vi "Ensemble Empirical Mode Decomposition.vi"(5 "Ensemble Size":u32, 7 "IMF Tolerance":dbl=0.2 format="%#_13g", 11 "Waveform":waveform(dbl)) -> (0 "df":dbl, 1 "dt":dbl, 2 "Hilbert Spectra":dbl[][][](array[numeric]), 3 "IMF Array":waveform(dbl)[](array[waveform]))   [LabVIEW 2013, in "Empirical Mode Decomposition.lvlib"]
uses:
  Empirical Mode Decomposition.lvlib
  <vilib>/Waveform/WDTOps.llb/WDT Number of Waveform Samples DBL.vi
  <vilib>/measure/mascope.llb/Amplitude and Levels 1 chan.vi
  <vilib>/measure/NI_MABase.lvlib
  <vilib>/measure/NI_MAPro.lvlib
  Popup Progress Bar/Popup Progress Bar.lvlib
panel:
  out "IMF + 0":waveform(dbl)[](graph)
  out "IMF":waveform(dbl)[](graph)
  # "TODO: Smooth out the Hilbert Spectrum graph"
  # "Scale                  Index\n1                              512-1023\n2                              256-511\n3                              128-255\n4                              64-127\n5                              32-63\n6                              16-31\n7                              8-15\n8                              4-7\n9                              2-3"
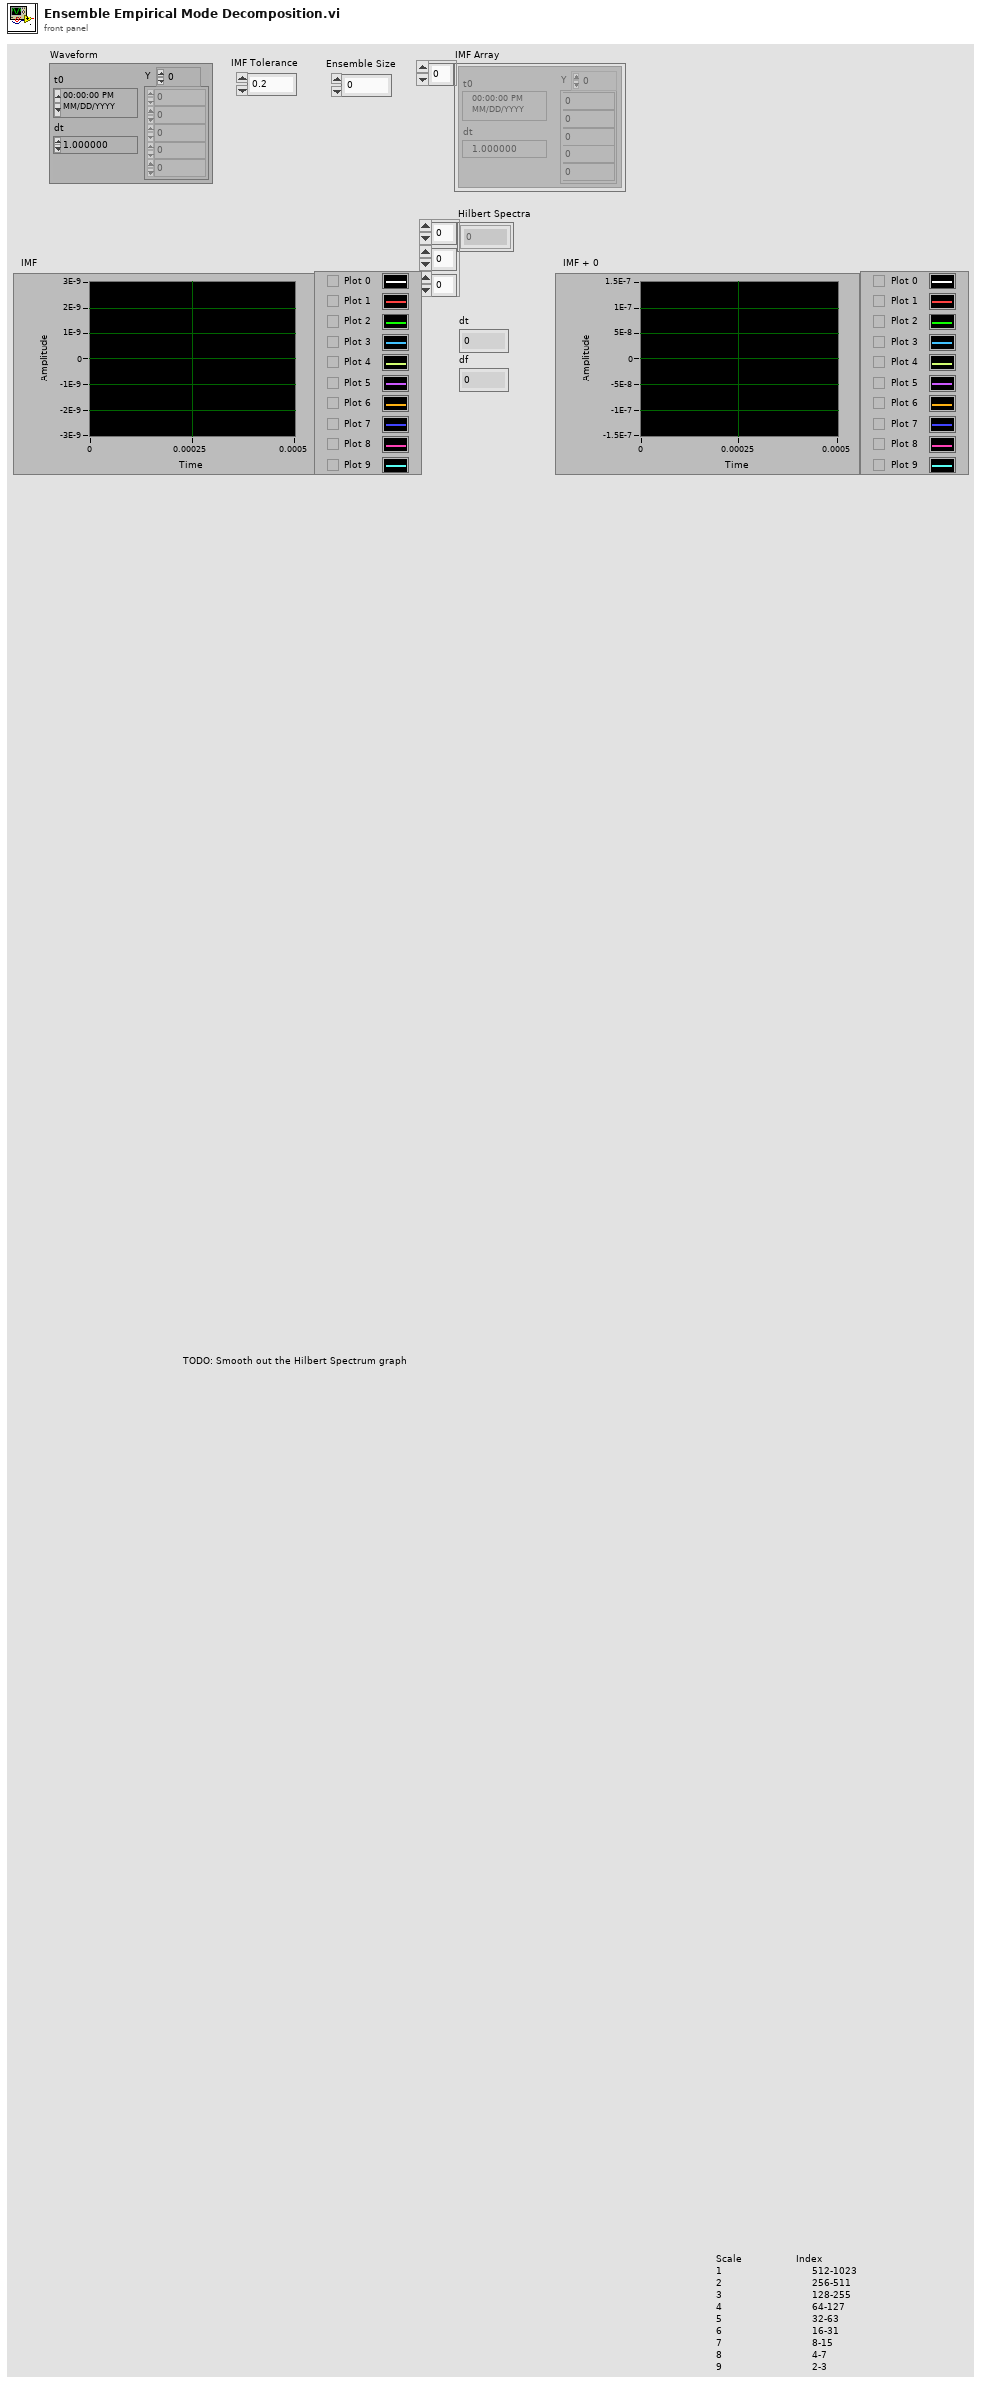
[diagram p1: front panel]
types:
  T1 = cluster{"This VI":refnum<vi>, "notifier out":refnum<notifier>}
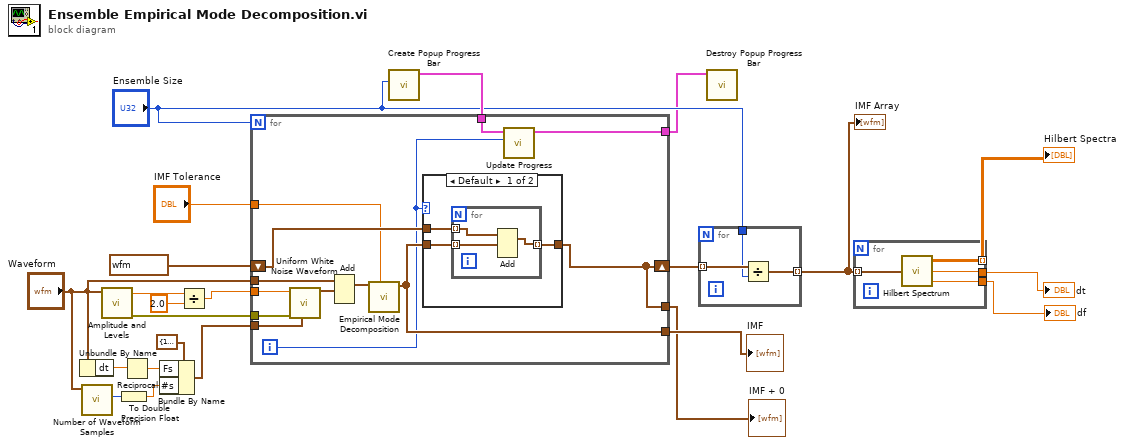
[diagram p0: block diagram]
diagram:
  n1 = Unbundle By Name("Waveform") -> ("dt"=w16:dbl)
  n2 = call-poly <vilib>:"Number of Waveform Samples.vi"("waveform in"="Waveform") -> ("number of samples"=w12:i32)  [unwired: 8 in, 2 out]
  n3 = call-poly <vilib>:"Amplitude and Levels.vi"("signal in"="Waveform") -> ("error out"=w23:errorcluster, "amplitude"=w7:dbl)  [unwired: 7 in, 2 out]
  n4 = To Double Precision Float(number=w12) -> (double precision float=w13:dbl)
  n5 = Reciprocal(x=w16) -> (1/x=w14:dbl)
  n6 = Bundle By Name(cluster=cluster{"Fs":dbl, "#s":dbl} {"Fs"=1000.0, "#s"=1000.0} ("sampling info"), "Fs"=w14, "#s"=w13) -> (w11:cluster{"Fs":dbl, "#s":dbl})
  n7 = Divide(x=w7, y=2.0) -> (x/y=w5:dbl)
  n8 = call "Create Popup Progress Bar.vi"("100% Value (100)"="Ensemble Size") -> ("bar ref"=w3:T1)  [unwired: 9 in, 1 out]
  n9 = for {
    N: "Ensemble Size" -> [_]
    tunnel: w5 -> [w36]
    tunnel: w23 -> [w35]
    tunnel: "Waveform" -> [w33]
    shift-right: [w28] -> w21
    shift-left: waveform(dbl)[] [{"t0"=timestamp(3516206484.2410417 s since 1904-01-01), "dt"=2e-12, "Y"=array[251 elements]}, {"t0"=timestamp(3516206484.2410417 s since 1904-01-01), "dt"=2e-12, "Y"=array[251 elements]}, {"t0"=timestamp(3516206484.2410417 s since 1904-01-01), "dt"=2e-12, "Y"=array[251 elements]}] ("IMF Array") -> [w29]
    tunnel: w11 -> [w31]
    tunnel: [w28] -> w8
    tunnel: [w30] -> w9
    tunnel: "IMF Tolerance" -> [w27]
    tunnel: w3 -> [w26]
    tunnel: [w24] -> w1
    i -> [w25]
    n10 = call <vilib>:"Uniform White Noise Waveform.vi"("sampling info"=w31, "error in (no error)"=w35, "amplitude"=w36) -> ("signal out"=w34:waveform(dbl))  [unwired: 7 in, 1 out]
    n11 = Add(1:w34, 2:w33) -> (0:w32:waveform(dbl))  [unwired: 1 in, 1 out]
    n12 = call "Empirical Mode Decomposition.vi"("IMF Tolerance"=w27, "Waveform"=w32) -> ("IMF Array"=w30:waveform(dbl)[])  [unwired: 6 in, 3 out]
    n13 = case shown="Default" w25 {
      tunnel: w30 -> [w39 w43]
      tunnel: [w37 w43] -> w28
      tunnel: w29 -> [w38 _]
      frame Default {
        n14 = for {
          tunnel: w39 -> [w41] mode=indexing
          tunnel: w38 -> [w42] mode=indexing
          tunnel: [w40] -> w37 mode=indexing
          n15 = Add(1:w41, 2:w42) -> (0:w40:waveform(dbl))  [unwired: 1 in, 1 out]
        }
      }
      frame 0 {
      }
    }
    n16 = call "Update Progress.vi"("Value"=w25, "bar ref in"=w26) -> ("bar ref out"=w24:T1)  [unwired: 8 in, 1 out]
  }
  "IMF" <- w9
  "IMF + 0" <- w8
  n17 = for {
    tunnel: w21 -> [w46] mode=indexing
    tunnel: [w45] -> w20 mode=indexing
    tunnel: "Ensemble Size" -> [w44]
    n18 = Divide(x=w46, y=w44) -> (x/y=w45:waveform(dbl))
  }
  "IMF Array" <- w20
  n19 = call "Destroy Popup Progress Bar.vi"("bar ref"=w1) -> ()  [unwired: 10 in, 1 out]
  n20 = for {
    tunnel: w20 -> [w50] mode=indexing
    tunnel: [w49] -> w19 mode=indexing
    tunnel: [w48] -> w18
    tunnel: [w47] -> w17
    n21 = call "Hilbert Spectrum.vi"("Waveform"=w50) -> ("df"=w47:dbl, "dt"=w48:dbl, "Spectrum"=w49:dbl[][])  [unwired: 2 in]
  }
  "Hilbert Spectra" <- w19
  "dt" <- w18
  "df" <- w17
